vi "Settings Dialog.vi"(8 "error in (no error)":errorcluster, 11 "Settings in":T5={"Support"={"Save Configuration"={"Log File Base Path"=path "", "TDMS File Reference"=refnum, "Reset"=FALSE, "Wait"=0.0, "Start Time"=0.0, "Update Rate"=1, "Channel Names"=[], "System Preset"=variant}, "LOG Configuration"={"LOG REF"=refnum, "Writer Queue"=refnum, "Log Path"=path "", "LOG"=FALSE}, "ALARM Configuration"={"LOG REF"=refnum, "Writer Queue"=refnum, "Log Path"=path "", "UPS standby"=FALSE, "status code"=5001, "SP"=[], "Over Sens Status"=[]}, "User Details"=[], "Radome Type"="", "Timer Configuration"={"Wait"=0.0, "Next Step"="", "Writer Queue"=refnum, "Reset"=FALSE, "VISA resource"="", "Status"=[], "Valve Time"=[], "Timer queue"=refnum, "Current valve"=0, "Enable"=FALSE}}, "Process"={"Test Configuration"={"current Step"=0, "Wait"=0.0, "Next Step"="", "Writer Queue"=refnum, "Reset"=FALSE, "SEQ Time"=0, "General Reset"=FALSE, "Cycles"=0, "Status"=[], "Ready"=[], "Backward"=FALSE, "Current SP"=[], "System Preset"={"Test Configuration"={"Cycles"=0, "Z Up"=0.0, "SP List"=[], "Operator"="", "Point Delay"=0, "Z Up 2"=0.0, "Cleaning In"=0.0, "Cleaning Out"=0.0, "Cleaning Cycles"=0}, "Test_Start_date"=""}, "Test Type"=enum."Calibration", "Sample Count"=0, "Local Queues"={"Cycles queue"=refnum, "Step queue"=refnum, "RES Queue"=refnum, "Clean queue"=refnum, "PS Scan queue"=refnum}, "current Clean"=0, "PS Measure Plan"=[]}}, "Report Configuration"={"Test Setting"={"Test_Num"=0, "Test_ID"=0, "Proc_ID"=0, "Max Force"=0.0, "User"="", "SN"="", "Date"=""}, "Measurements"=[], "LOG REF"=refnum, "Report Template"=path "", "Save Report path"=path "", "Data File Path"=path "", "Popup Dialog"=FALSE}, "History Data"={"Tests"=[], "Test Name"=""}, "Motor Configuration"={"Tango HW"={"VISA resource"="", "Baud Rate (115200)"=2, "lAnInterfaceType"=0, "bAShowProt"=15}, "Writer Queue"=refnum, "Status"=FALSE, "Abs Position"=[], "Axis Velocity"={"dX"=0.0, "dY"=0.0, "dZ"=0.0, "dA"=0.0}, "acceleration "=0.0, "Z direction"=enum."Up", "Position Mode"="", "plLSID"=0}, "PalmSense  Configuration"={"PalmSens.lvclass"=refnum, "Writer Queue"=refnum, "Enable"=FALSE, "Is Measuring Ref"=refnum, "Method"={"Name"="", "Method Ref"=variant}, "PS Live Curve Result"=refnum}, "Hiden Scanner Resources"={"Link"={"Connection"=enum."USB", "Host or IP address (TCP/IP)"="", "Port (Serial/USB)"="COM1"}, "VISA resource"="", "Writer Queue"=refnum, "Status"=FALSE}, "MFC Configuration"={"MFC Definition"={"MFC Port"="", "MFC Enable"=TRUE, "Baud Rate"=0, "Interface type"=enum."RS-485", "Address"=0}, "Set Point Options"={"Setpoint Value"=0.0, "Mass Flow EU 2"="", "Setpoint Source"="", "Valve Mode"=""}, "Writer Queue"=refnum, "Enable"=FALSE, "Update Rate"=0, "MRC Chamber Enable"=FALSE, "Selected Gas"="", "Address String"=""}, "Pump Configuration"={"Pump  name"=[], "Writer Queue"=refnum, "Pump Info"={"Pump Type"="", "Speed"=0, "Direction"=0, "Running"=FALSE}, "Current Pump Name"="", "Wait"=0.0, "Next Step"="", "Reset"=FALSE}} {"Pump Configuration"."Pump Info"."Direction" items=["CW", "CCW"]; "Pump Configuration"."Pump Info"."Speed" format="%03.0f"; "MFC Configuration"."Set Point Options"."Setpoint Value" min=0.0 max=0.62495 format="%.5f"; "Process"."Test Configuration"."PS Measure Plan" items=["Pretreatment settings (PS)", "Linear Sweep Voltammetry (LSV)", "Differential Pulse Voltammetry (DPV)", "Cyclic Voltammetry (CV)", "Chronoamperometry (CA)", "Chronopotentiometry (CP)", "El Imp Spectroscopy (EIS)"]; "Process"."Test Configuration"."System Preset"."Test Configuration"."SP List" format="%#.1g"; "Support"."Save Configuration"."Update Rate" min=1 max=10 step=1}) -> (0 "error out":errorcluster, 1 "Cancelled?":bool, 2 "UI Refresh Needed?":bool, 3 "Settings out":T5={"Support"={"Save Configuration"={"Log File Base Path"=path "", "TDMS File Reference"=refnum, "Reset"=FALSE, "Wait"=0.0, "Start Time"=0.0, "Update Rate"=1, "Channel Names"=[], "System Preset"=variant}, "LOG Configuration"={"LOG REF"=refnum, "Writer Queue"=refnum, "Log Path"=path "", "LOG"=FALSE}, "ALARM Configuration"={"LOG REF"=refnum, "Writer Queue"=refnum, "Log Path"=path "", "UPS standby"=FALSE, "status code"=5001, "SP"=[], "Over Sens Status"=[]}, "User Details"=[], "Radome Type"="", "Timer Configuration"={"Wait"=0.0, "Next Step"="", "Writer Queue"=refnum, "Reset"=FALSE, "VISA resource"="", "Status"=[], "Valve Time"=[], "Timer queue"=refnum, "Current valve"=0, "Enable"=FALSE}}, "Process"={"Test Configuration"={"current Step"=0, "Wait"=0.0, "Next Step"="", "Writer Queue"=refnum, "Reset"=FALSE, "SEQ Time"=0, "General Reset"=FALSE, "Cycles"=0, "Status"=[], "Ready"=[], "Backward"=FALSE, "Current SP"=[], "System Preset"={"Test Configuration"={"Cycles"=0, "Z Up"=0.0, "SP List"=[], "Operator"="", "Point Delay"=0, "Z Up 2"=0.0, "Cleaning In"=0.0, "Cleaning Out"=0.0, "Cleaning Cycles"=0}, "Test_Start_date"=""}, "Test Type"=enum."Calibration", "Sample Count"=0, "Local Queues"={"Cycles queue"=refnum, "Step queue"=refnum, "RES Queue"=refnum, "Clean queue"=refnum, "PS Scan queue"=refnum}, "current Clean"=0, "PS Measure Plan"=[]}}, "Report Configuration"={"Test Setting"={"Test_Num"=0, "Test_ID"=0, "Proc_ID"=0, "Max Force"=0.0, "User"="", "SN"="", "Date"=""}, "Measurements"=[], "LOG REF"=refnum, "Report Template"=path "", "Save Report path"=path "", "Data File Path"=path "", "Popup Dialog"=FALSE}, "History Data"={"Tests"=[], "Test Name"=""}, "Motor Configuration"={"Tango HW"={"VISA resource"="", "Baud Rate (115200)"=2, "lAnInterfaceType"=0, "bAShowProt"=15}, "Writer Queue"=refnum, "Status"=FALSE, "Abs Position"=[], "Axis Velocity"={"dX"=0.0, "dY"=0.0, "dZ"=0.0, "dA"=0.0}, "acceleration "=0.0, "Z direction"=enum."Up", "Position Mode"="", "plLSID"=0}, "PalmSense  Configuration"={"PalmSens.lvclass"=refnum, "Writer Queue"=refnum, "Enable"=FALSE, "Is Measuring Ref"=refnum, "Method"={"Name"="", "Method Ref"=variant}, "PS Live Curve Result"=refnum}, "Hiden Scanner Resources"={"Link"={"Connection"=enum."USB", "Host or IP address (TCP/IP)"="", "Port (Serial/USB)"="COM1"}, "VISA resource"="", "Writer Queue"=refnum, "Status"=FALSE}, "MFC Configuration"={"MFC Definition"={"MFC Port"="", "MFC Enable"=TRUE, "Baud Rate"=0, "Interface type"=enum."RS-485", "Address"=0}, "Set Point Options"={"Setpoint Value"=0.0, "Mass Flow EU 2"="", "Setpoint Source"="", "Valve Mode"=""}, "Writer Queue"=refnum, "Enable"=FALSE, "Update Rate"=0, "MRC Chamber Enable"=FALSE, "Selected Gas"="", "Address String"=""}, "Pump Configuration"={"Pump  name"=[], "Writer Queue"=refnum, "Pump Info"={"Pump Type"="", "Speed"=0, "Direction"=0, "Running"=FALSE}, "Current Pump Name"="", "Wait"=0.0, "Next Step"="", "Reset"=FALSE}} {"Pump Configuration"."Pump Info"."Direction" items=["CW", "CCW"]; "Pump Configuration"."Pump Info"."Speed" format="%03.0f"; "MFC Configuration"."Set Point Options"."Setpoint Value" min=0.0 max=0.62495 format="%.5f"; "Process"."Test Configuration"."PS Measure Plan" items=["Pretreatment settings (PS)", "Linear Sweep Voltammetry (LSV)", "Differential Pulse Voltammetry (DPV)", "Cyclic Voltammetry (CV)", "Chronoamperometry (CA)", "Chronopotentiometry (CP)", "El Imp Spectroscopy (EIS)"]; "Process"."Test Configuration"."System Preset"."Test Configuration"."SP List" format="%#.1g"; "Support"."Save Configuration"."Update Rate" min=1 max=10 step=1})   [LabVIEW 2020, in "Settings.lvlib"]
doc: "Dialog for selecting user specified settings."
uses:
  Settings.lvlib
  Settings.ctl
  <instrlib>/PalmSens SDK for LabVIEW 5.10/PalmSens/PalmSens.lvclass
  Logging/Save Configuration.ctl
  LOG/LOG Configuration.ctl
  support/Message Queue/Message Cluster.ctl
  ALARM/ALARM Configuration.ctl
  Valve Control/AM Configuration.ctl
  Test Driver/Test Driver Configuration.ctl
  Test Driver/System Preset.ctl
  Test Driver/Test Type.ctl
  Report/REP Configuration.ctl
  Report/Test Setting.ctl
  MOTOR/PS Hardware Configuration.ctl
  DMM/PalmSense Hardware Configuration.ctl
  Hiden Scanner/Scanner Hardware Configuration.ctl
  MRC/MRC Configuration.ctl
  WM Pump/Pump Hardware Configuration.ctl
  support/PCT FGV CMD.ctl
  <vilib>/Utility/file.llb/Write Delimited Spreadsheet (DBL).vi
  <vilib>/Utility/file.llb/Read Delimited Spreadsheet (DBL).vi
  <vilib>/Analysis/1siggen.llb/Ramp Pattern by Delta.vi
  <vilib>/gmath/interp.llb/Create Mesh Grid (2D) (x,y arrays).vi
  <vilib>/Utility/xml.llb/Write to XML File(string).vi
  <vilib>/Analysis/NI_AALBase.lvlib
  <vilib>/gmath/NI_Gmath.lvlib
  Logging/SAVE.lvlib
  support/Message Queue/Message Queue.lvlib
  LOG/LOG.lvlib
  ALARM/QCT ALARM.lvlib
  Report/Report.lvlib
  MOTOR/MOTOR.lvlib
  Test Driver/Test Driver.lvlib
  DMM/PalmSens.lvlib
  Hiden Scanner/Hiden Scanner.lvlib
  Valve Control/Valve Control.lvlib
  MRC/MRC Module.lvlib
  WM Pump/Pump.lvlib
panel:
  in  "OK Button":bool
  in  "Cancel Button":bool
  out "Tab Control":enum32{"Administrator", "System", "Test"}(tab)
  in  "Tango XYZ":T1={"Position Mode"="Absolute", "XYZ Velocity"=0.0}
  in  "PS Measure Plan":u16[](array[ring]) items=["Pretreatment settings (PS)", "Linear Sweep Voltammetry (LSV)", "Differential Pulse Voltammetry (DPV)", "Cyclic Voltammetry (CV)", "Chronoamperometry (CA)", "Chronopotentiometry (CP)", "El Imp Spectroscopy (EIS)"]
  in  "Hiden Scan Details":dbl[][](array[numeric])=[[28.0, 28.0]]
  in  "PS Measure Type List":u16(ring)=1 items=["Pretreatment settings (PS)", "Linear Sweep Voltammetry (LSV)", "Differential Pulse Voltammetry (DPV)", "Cyclic Voltammetry (CV)", "Chronoamperometry (CA)", "Chronopotentiometry (CP)", "El Imp Spectroscopy (EIS)"]
  in  "Log File Path":path
  in  "Save Report Path":path
  in  "Report Template":path
  in  "Hiden Input details":T2={"Input device"="Faraday", "Autorange High"=-7, "Autorange Low"=-7, "Start range"=-7, "Dwell (%)"=100, "Settle (%)"=100, "Dwell is ms?"=FALSE, "Settle is ms?"=FALSE}
  out "Technician":string
  in  "Main Axis":enum32{"X Axis", "Y Axis"}(radio)
  in  "Square":cluster{"Start":dbl, "End":dbl, "delta":dbl} caption="Square / Radius SET"
  in  "Circle":cluster{"Points N":dbl, "M Point":dbl[]} caption="Y Start-Stop Point"
  in  "Shape Type":T3(ring)
  in  "Test Configuration":T4 {"SP List" format="%#.1g"}
  in  "Tests List":string(combo)
  in  "Save Test":bool
  out "XY Graph":cluster{"X":dbl[], "Y":dbl[]}[](graph)
  in  "Radio Buttons":enum32{"Administrator", "System", "Test"}(radio)=enum."System"
  out "power":bool
  # "Non visible portion of dialog (needed for connector pane)."
  # "TANGO XYZ"
  # "X"
  # "Y"
  # "Cycles"
  # "Point Delay"
  # "Up"
  # "Down"
  # "Z Axes"
  # "#C"
  # "In"
  # "Out"
  # "Cleaning [sec]"
  # "X"
  # "Y"
  # "Cycles"
  # "Point Delay"
  # "Up"
  # "Down"
  # "Z Axes"
  # "#C"
  # "In"
  # "Out"
  # "Cleaning [sec]"
  # "X"
  # "Y"
  # "Cycles"
  # "Point Delay"
  # "Up"
  # "Down"
  # "Z Axes"
  # "#C"
  # "In"
  # "Out"
  # "Cleaning [sec]"
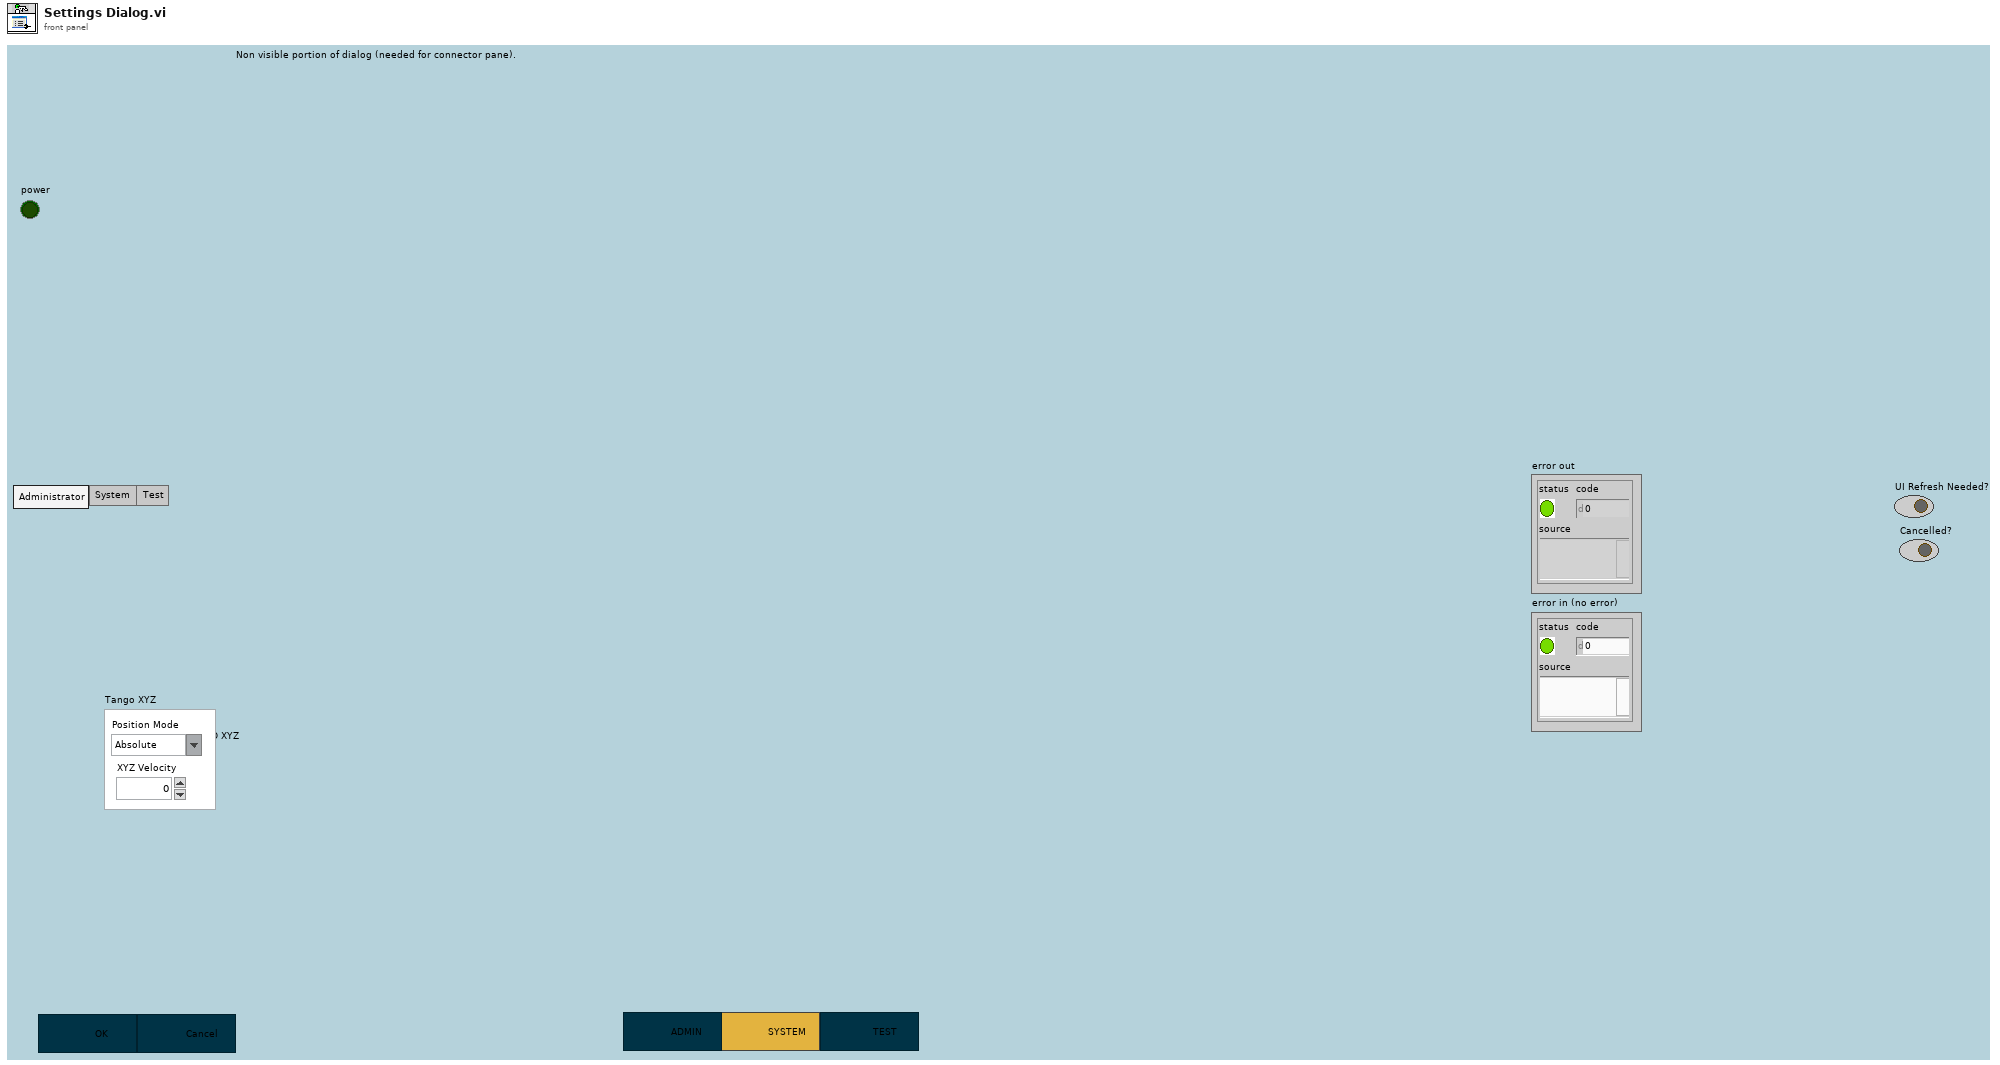
[diagram p1: front panel]
types:
  T1 = cluster{"Position Mode":string, "XYZ Velocity":dbl}
  T2 = cluster{"Input device":string, "Autorange High":i16, "Autorange Low":i16, "Start range":i16, "Dwell (%)":u16, "Settle (%)":u16, "Dwell is ms?":bool, "Settle is ms?":bool}
  T3 = enum16{"Circle", "Square", "Ramp", "Mesh", "Line"}
  T4 = cluster{"Cycles":i32, "Z Up":dbl, "SP List":dbl[][], "Operator":string, "Point Delay":i32, "Z Up 2":dbl, "Cleaning In":dbl, "Cleaning Out":dbl, "Cleaning Cycles":i32}
  T5 = typedef "Settings.lvlib/Settings.ctl" = cluster{"Support":cluster{"Save Configuration":T6, "LOG Configuration":T7, "ALARM Configuration":T8, "User Details":string[], "Radome Type":string, "Timer Configuration":T9}, "Process":cluster{"Test Configuration":T10}, "Report Configuration":T13, "History Data":cluster{"Tests":string[][], "Test Name":string}, "Motor Configuration":T15, "PalmSense  Configuration":T16, "Hiden Scanner Resources":T17, "MFC Configuration":T18, "Pump Configuration":T19}
  T6 = typedef "SAVE.lvlib/Save Configuration.ctl" = cluster{"Log File Base Path":path, "TDMS File Reference":refnum<k34>, "Reset":bool, "Wait":dbl, "Start Time":dbl, "Update Rate":u16, "Channel Names":string[], "System Preset":variant}
  T7 = typedef "LOG.lvlib/LOG Configuration.ctl" = cluster{"LOG REF":refnum<vi>, "Writer Queue":refnum<queue>, "Log Path":path, "LOG":bool}
  T8 = typedef "QCT ALARM.lvlib/ALARM Configuration.ctl" = cluster{"LOG REF":refnum<vi>, "Writer Queue":refnum<queue>, "Log Path":path, "UPS standby":bool, "status code":i32, "SP":dbl[], "Over Sens Status":dbl[]}
  T9 = typedef "Valve Control.lvlib/AM Configuration.ctl" = cluster{"Wait":dbl, "Next Step":string, "Writer Queue":refnum<queue>, "Reset":bool, "VISA resource":refnum<visa-resource-name>, "Status":bool[], "Valve Time":dbl[], "Timer queue":refnum<queue>, "Current valve":i32, "Enable":bool}
  T10 = typedef "Test Driver.lvlib/Test Driver Configuration.ctl" = cluster{"current Step":i32, "Wait":dbl, "Next Step":string, "Writer Queue":refnum<queue>, "Reset":bool, "SEQ Time":i32, "General Reset":bool, "Cycles":i32, "Status":bool[], "Ready":bool[], "Backward":bool, "Current SP":dbl[], "System Preset":T11, "Test Type":T12, "Sample Count":i32, "Local Queues":cluster{"Cycles queue":refnum<queue>, "Step queue":refnum<queue>, "RES Queue":refnum<queue>, "Clean queue":refnum<queue>, "PS Scan queue":refnum<queue>}, "current Clean":i32, "PS Measure Plan":u16[]}
  T11 = typedef "System Preset.ctl" = cluster{"Test Configuration":cluster{"Cycles":i32, "Z Up":dbl, "SP List":dbl[][], "Operator":string, "Point Delay":i32, "Z Up 2":dbl, "Cleaning In":dbl, "Cleaning Out":dbl, "Cleaning Cycles":i32}, "Test_Start_date":string}
  T12 = typedef "Test Driver.lvlib/Test Type.ctl" = enum16{"Calibration", "Test"}
  T13 = typedef "Report.lvlib/REP Configuration.ctl" = cluster{"Test Setting":T14, "Measurements":string[][], "LOG REF":refnum<vi>, "Report Template":path, "Save Report path":path, "Data File Path":path, "Popup Dialog":bool}
  T14 = typedef "Report.lvlib/Test Setting.ctl" = cluster{"Test_Num":i32, "Test_ID":i32, "Proc_ID":i32, "Max Force":dbl, "User":string, "SN":string, "Date":string}
  T15 = typedef "MOTOR.lvlib/PS Hardware Configuration.ctl" = cluster{"Tango HW":cluster{"VISA resource":refnum<visa-resource-name>, "Baud Rate (115200)":i32, "lAnInterfaceType":i32, "bAShowProt":i32}, "Writer Queue":refnum<queue>, "Status":bool, "Abs Position":i32[], "Axis Velocity":cluster{"dX":dbl, "dY":dbl, "dZ":dbl, "dA":dbl}, "acceleration ":dbl, "Z direction":enum16{"Up", "Down"}, "Position Mode":string, "plLSID":i32}
  T16 = typedef "PalmSens.lvlib/PalmSense Hardware Configuration.ctl" = cluster{"PalmSens.lvclass":refnum<class "PalmSens.lvclass">, "Writer Queue":refnum<queue>, "Enable":bool, "Is Measuring Ref":refnum<vi>, "Method":cluster{"Name":string, "Method Ref":variant}, "PS Live Curve Result":refnum<vi>}
  T17 = typedef "Hiden Scanner.lvlib/Scanner Hardware Configuration.ctl" = cluster{"Link":cluster{"Connection":enum16{"Serial", "TCP/IP", "USB"}, "Host or IP address (TCP/IP)":string, "Port (Serial/USB)":string}, "VISA resource":refnum<visa-resource-name>, "Writer Queue":refnum<queue>, "Status":bool}
  T18 = typedef "MRC Module.lvlib/MRC Configuration.ctl" = cluster{"MFC Definition":cluster{"MFC Port":refnum<visa-resource-name>, "MFC Enable":bool, "Baud Rate":i32, "Interface type":enum32{"RS-485", "RS-232"}, "Address":i32}, "Set Point Options":cluster{"Setpoint Value":dbl, "Mass Flow EU 2":string, "Setpoint Source":string, "Valve Mode":string}, "Writer Queue":refnum<queue>, "Enable":bool, "Update Rate":u32, "MRC Chamber Enable":bool, "Selected Gas":string, "Address String":string}
  T19 = typedef "Pump.lvlib/Pump Hardware Configuration.ctl" = cluster{"Pump  name":refnum<visa-resource-name>[], "Writer Queue":refnum<queue>, "Pump Info":cluster{"Pump Type":string, "Speed":i32, "Direction":u16, "Running":bool}, "Current Pump Name":refnum<visa-resource-name>, "Wait":dbl, "Next Step":string, "Reset":bool}
  T20 = typedef "PCT FGV CMD.ctl" = enum16{"INIT", "GET", "SET"}
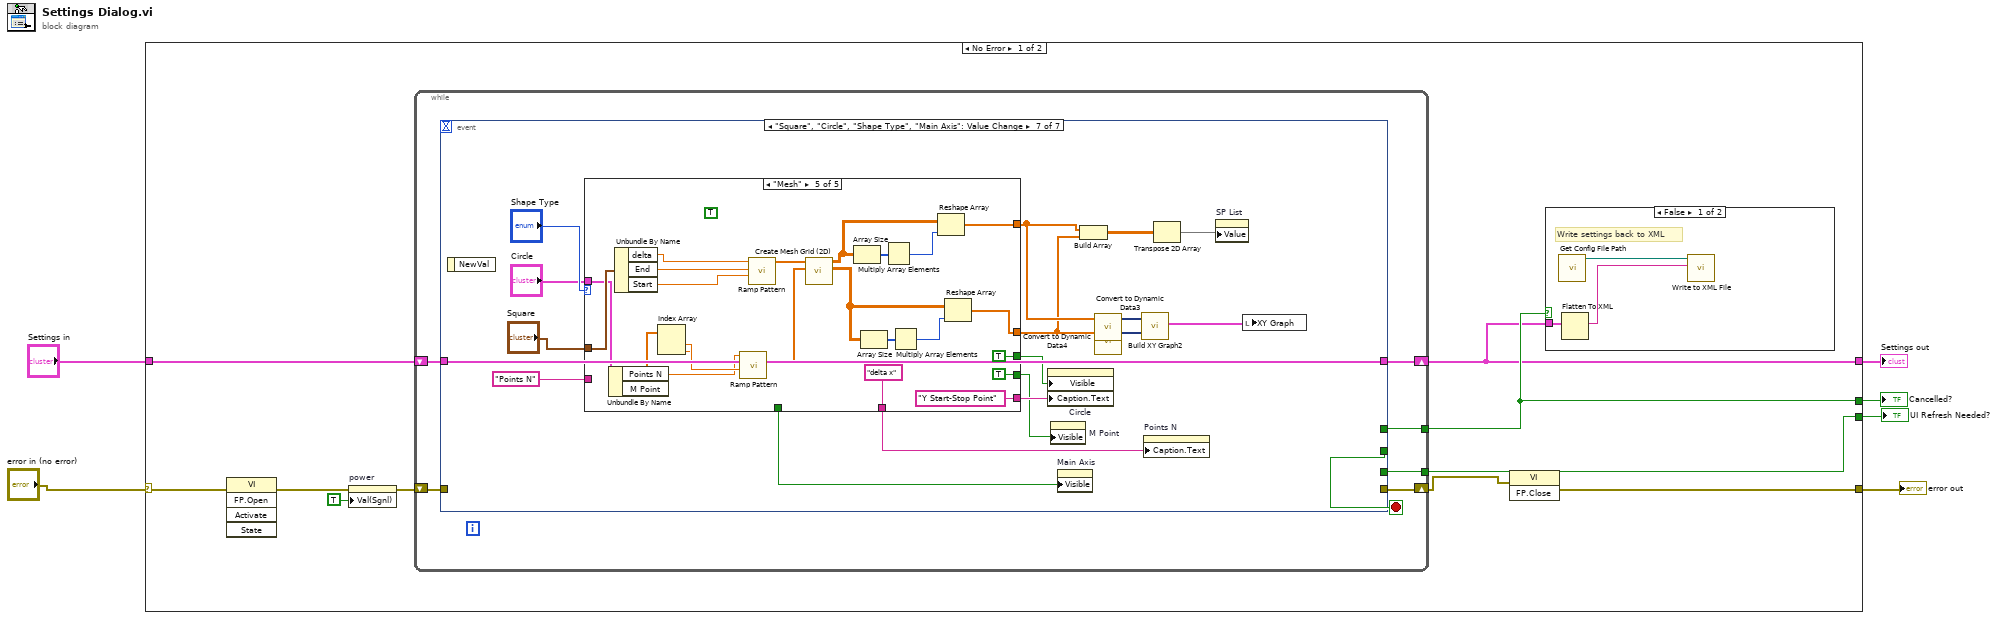
[diagram p0: block diagram]
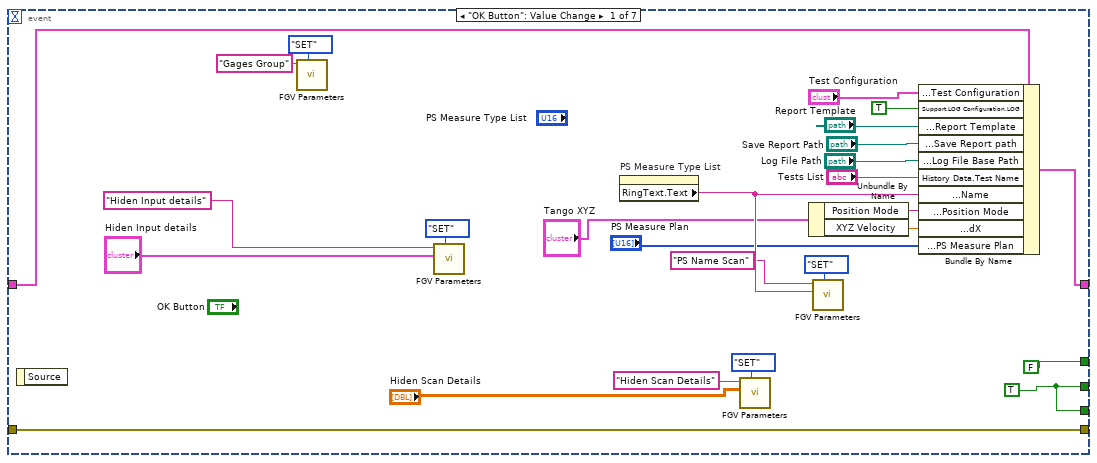
[diagram p2: hidden frame]
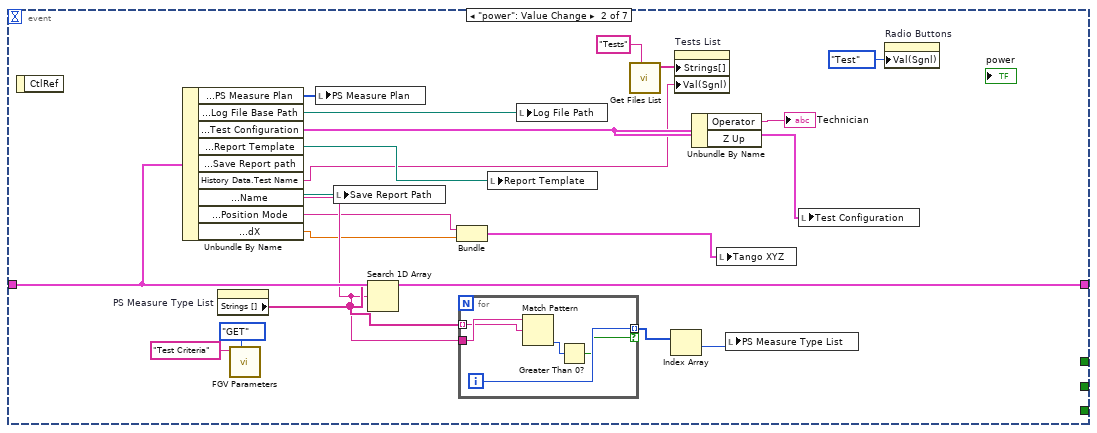
[diagram p3: hidden frame]
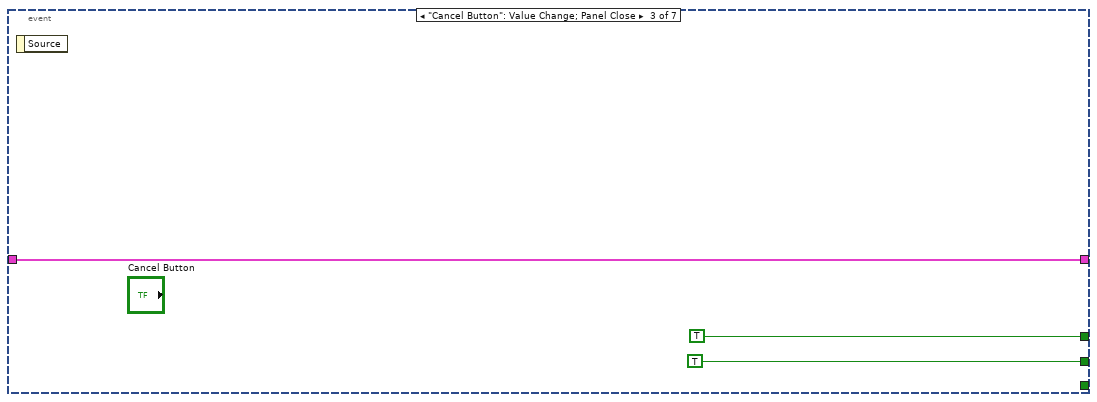
[diagram p4: hidden frame]
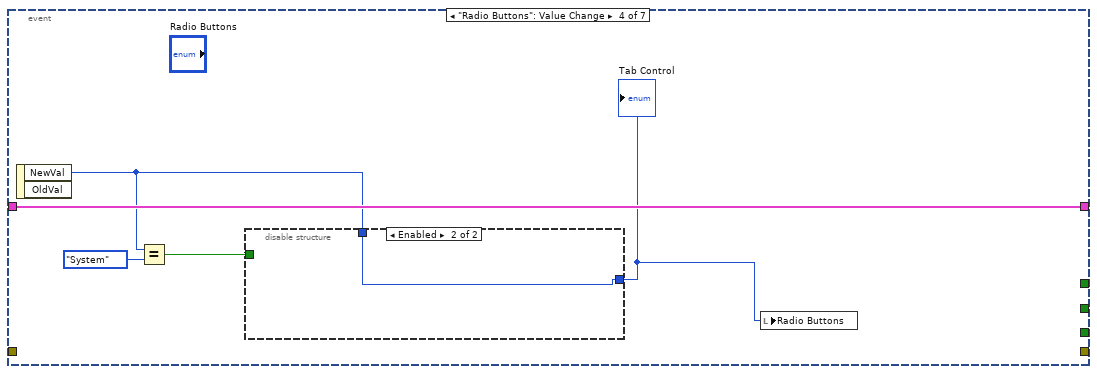
[diagram p5: hidden frame]
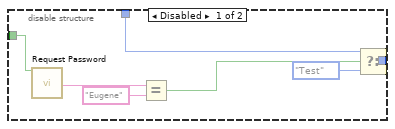
[diagram p6: hidden frame]
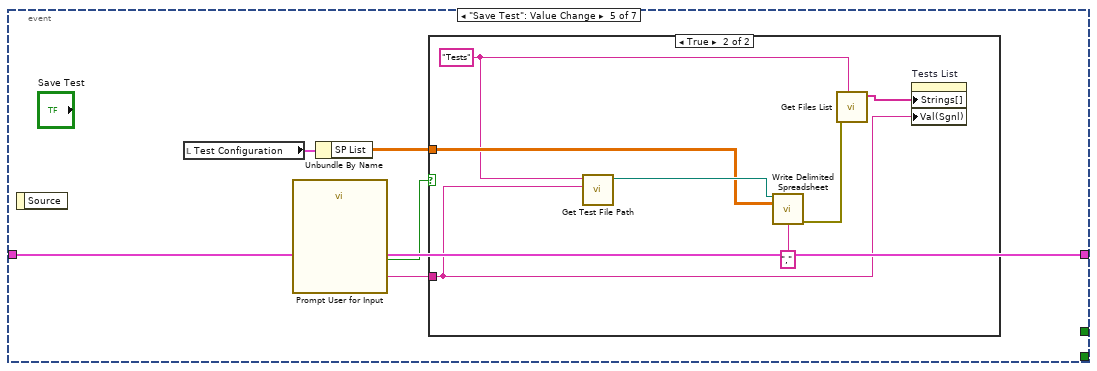
[diagram p7: hidden frame]
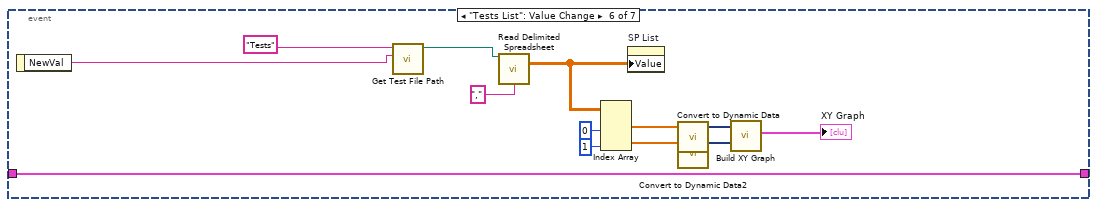
[diagram p9: hidden frame]
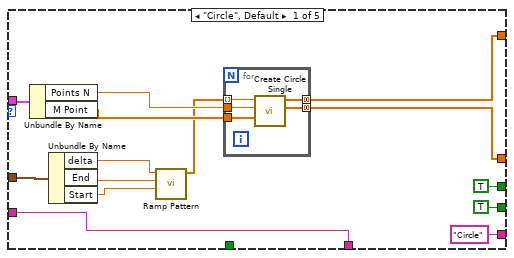
[diagram p10: hidden frame]
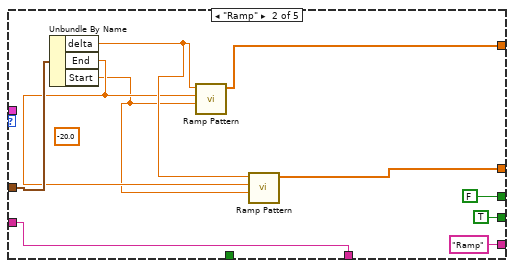
[diagram p11: hidden frame]
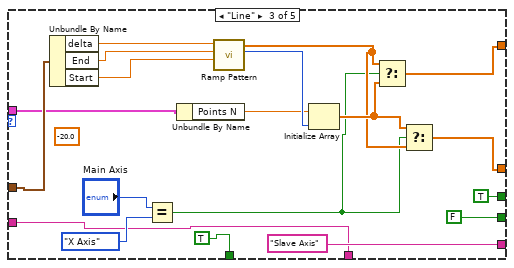
[diagram p12: hidden frame]
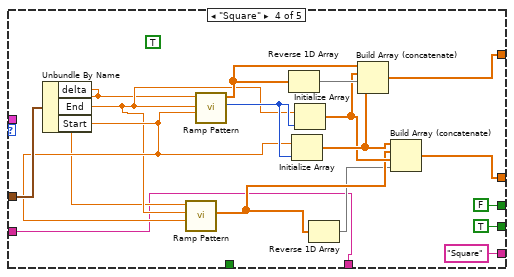
[diagram p13: hidden frame]
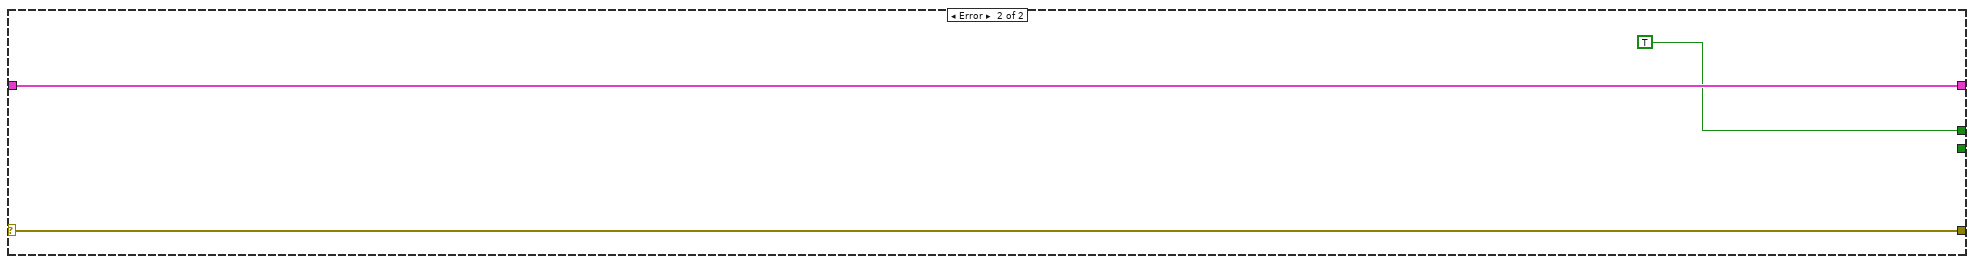
[diagram p15: hidden frame]
diagram:
  n1 = case shown="No Error" "error in (no error)" {
    selector: "error in (no error)" -> [w12 w226]
    tunnel: [w11 w226] -> w5
    tunnel: "Settings in" -> [w14 w225]
    tunnel: [w15 w225] -> w4
    tunnel: [w7 _] -> w3
    tunnel: [w16 TRUE ("UI Refresh Needed?")] -> w2
    frame No Error {
      n2 = invoke class="VI" method="FP.Open"(error in=w12) -> (error out=w10:errorcluster)  [unwired: 4 in, 4 out]
      n3 = property on="power" class="Bool (strict)"(error in=w10, "Val(Sgnl)"=TRUE ("Value (Signaling)")) -> (error out=w8:errorcluster)  [unwired: 1 in, 1 out]
      n4 = while {
        tunnel: [w19] -> w16
        shift-right: [w23] -> w15
        shift-left: w14 -> [w22]
        shift-right: [w20] -> w13
        shift-left: w8 -> [w21]
        tunnel: [w17] -> w7
        stop <- w18 stop-if-true
        n5 = event shown="[6] \"Square\", \"Circle\", \"Shape Type\", \"Main Axis\": Value Change" {
          selector: _ -> [_ _ _ _ _ _ _]
          dyn-events: _ -> [_ _ _ _ _ _ _]
          timeout: _ -> [_ _ _ _ _ _ _]
          tunnel: [w48 w69 w77 w82 w95 w115 w132] -> w23
          tunnel: w22 -> [w43 w69 w77 w82 w95 w115 w132]
          tunnel: [FALSE ("UI Refresh Needed?") _ TRUE ("UI Refresh Needed?") _ _ _ _] -> w19
          tunnel: w21 -> [w47 _ _ _ _ _ _]
          tunnel: [w47 _ _ _ _ _ _] -> w20
          tunnel: [w39 _ TRUE _ _ _ _] -> w18
          tunnel: [w39 _ _ _ _ _ _] -> w17
          event "OK Button": Value Change {
            w39 = TRUE
            n6 = event-data() -> ()  [unwired: 1 in, 1 out]
            n7 = call "FGV Parameters.vi"("CMD"=PCT_FGV_CMD."SET", "Key"="Gages Group") -> ()  [unwired: 7 in, 3 out]
            n8 = call "FGV Parameters.vi"("CMD"=PCT_FGV_CMD."SET", "input"="Hiden Input details", "Key"="Hiden Input details") -> ()  [unwired: 6 in, 3 out]
            n9 = property on="PS Measure Type List" class="Ring (strict)"() -> ("RingText.Text"=w29:string)  [unwired: 2 in, 2 out]
            n10 = call "FGV Parameters.vi"("CMD"=PCT_FGV_CMD."SET", "input"="Hiden Scan Details", "Key"="Hiden Scan Details") -> ()  [unwired: 6 in, 3 out]
            n11 = Unbundle By Name("Tango XYZ") -> ("Position Mode"=w27:string, "XYZ Velocity"=w25:dbl)
            n12 = call "FGV Parameters.vi"("CMD"=PCT_FGV_CMD."SET", "input"=w29, "Key"="PS Name Scan") -> ()  [unwired: 6 in, 3 out]
            n13 = Bundle By Name(cluster=w43, "Process.Test Configuration.System Preset.Test Configuration"="Test Configuration", "Support.LOG Configuration.LOG"=TRUE, "Report Configuration.Report Template"="Report Template", "Report Configuration.Save Report path"="Save Report Path", "Support.Save Configuration.Log File Base Path"="Log File Path", "History Data.Test Name"="Tests List", "PalmSense  Configuration.Method.Name"=w29, "Motor Configuration.Position Mode"=w27, "Motor Configuration.Axis Velocity.dX"=w25, "Process.Test Configuration.PS Measure Plan"="PS Measure Plan") -> (w48:T5)
          }
          event "power": Value Change {
            n14 = event-data() -> ()  [unwired: 1 in, 1 out]
            n15 = Unbundle By Name(w69) -> ("Process.Test Configuration.PS Measure Plan"=w50:u16[], "Support.Save Configuration.Log File Base Path"=w66:path, "Process.Test Configuration.System Preset.Test Configuration"=w62:T4, "Report Configuration.Report Template"=w68:path, "Report Configuration.Save Report path"=w67:path, "History Data.Test Name"=w59:string, "PalmSense  Configuration.Method.Name"=w57:string, "Motor Configuration.Position Mode"=w53:string, "Motor Configuration.Axis Velocity.dX"=w52:dbl)
            n16 = property on="PS Measure Type List" class="Ring (strict)"() -> ("Strings []"=w58:string[])  [unwired: 2 in, 2 out]
            n17 = call "FGV Parameters.vi"("CMD"=PCT_FGV_CMD."GET", "Key"="Test Criteria") -> ()  [unwired: 7 in, 3 out]
            n18 = local write "PS Measure Plan"(w50) -> ()
            n19 = local write "Save Report Path"(w67) -> ()
            n20 = Search 1D Array(1D array=w58, element=w57) -> ()  [unwired: 1 in, 1 out]
            n21 = Bundle("Position Mode"=w53, "dX"=w52) -> (w51:cluster{"Position Mode":string, "dX":dbl})  [unwired: 1 in]
            n22 = for {
              tunnel: w58 -> [w73] mode=indexing
              tunnel: w57 -> [w74]
              tunnel: [w72] -> w56 mode=indexing if=w70
              i -> [w72]
              n23 = Match Pattern(string=w74, regular expression=w73) -> (offset past match=w71:i32)  [unwired: 1 in, 3 out]
              n24 = Greater Than 0?(x=w71) -> (x > 0?=w70:bool)
            }
            n25 = local write "Report Template"(w68) -> ()
            n26 = local write "Log File Path"(w66) -> ()
            n27 = call "Get Files List.vi"("Folder Name"="Tests") -> ("List"=w60:string[])  [unwired: 9 in, 1 out]
            n28 = Index Array(array=w56) -> (element=w55:i32)  [unwired: 1 in]
            n29 = property on="Tests List" class="CmbBox"("Strings[]"=w60, "Val(Sgnl)"=w59) -> ()  [unwired: 2 in, 2 out]
            n30 = Unbundle By Name(w62) -> ("Operator"=→"Technician":string)  [unwired: 1 out]
            n31 = local write "Tango XYZ"(w51) -> ()
            n32 = local write "PS Measure Type List"(w55) -> ()
            n33 = local write "Test Configuration"(w62) -> ()
            n34 = property on="Radio Buttons" class="RadioBtnsControl (strict)"("Val(Sgnl)"=enum32{"Administrator", "System", "Test"}."Test" ("Value (Signaling)")) -> ()  [unwired: 2 in, 2 out]
          }
          event "Cancel Button": Value Change; Panel Close {
            n35 = event-data() -> ()  [unwired: 1 in, 1 out]
          }
          event "Radio Buttons": Value Change {
            n36 = event-data() -> ("NewVal"=w80:enum32{"Administrator", "System", "Test"})  [unwired: 1 in, 1 out]
            n37 = Equal?(x=w80, y=enum32{"System", "Test"}."System") -> (x = y?=w79:bool)
            n38 = disable-structure shown="Enabled" {
              disable-tunnel: w80 -> [w86 w90]
              disable-tunnel: w79 -> [w85 _]
              disable-tunnel: [w84 w90] -> w78
              frame Disabled {
                n39 = call "Request Password.vi"("Enable"=w85) -> ("Password"=w89:string)  [unwired: 16 in, 2 out]
                n40 = Equal?(x=w89, y="Eugene") -> (x = y?=w83:bool)
                n41 = Select(t=w86, s=w83, f=enum32{"System", "Test"}."Test" ("Radio Buttons")) -> (s? t:f=w84:u32)
              }
              frame Enabled {
              }
            }
            "Tab Control" <- w78
            n42 = local write "Radio Buttons"(w78) -> ()
          }
          event "Save Test": Value Change {
            n43 = event-data() -> ()  [unwired: 1 in, 1 out]
            n44 = local read "Test Configuration"() -> (w94:T4)
            n45 = call "Prompt User for Input"() -> ("Test Name"=w92:string, "OK"=w93:bool)  [unwired: 17 in, 1 out]
            n46 = Unbundle By Name(w94) -> ("SP List"=w91:dbl[][])
            n47 = case shown="True" w93 {
              tunnel: w92 -> [_ w96]
              tunnel: w91 -> [_ w101]
              frame False {
              }
              frame True {
                w99 = "Tests" ("Folder Name")
                n48 = call "Get Test File Path.vi"("Test Name"=w96, "Folder Name"=w99) -> ("test path"=w102:path)  [unwired: 9 in]
                n49 = call-poly <vilib>:"Write Delimited Spreadsheet.vi"("file path (dialog if empty)"=w102, "2D data"=w101, "delimiter (\\t)"="," ("delimiter (\\t)")) -> ("error out"=w98:errorcluster)  [unwired: 11 in, 1 out]
                n50 = call "Get Files List.vi"("Folder Name"=w99, "error in (no error)"=w98) -> ("List"=w97:string[])  [unwired: 8 in, 1 out]
                n51 = property on="Tests List" class="CmbBox"("Strings[]"=w97, "Val(Sgnl)"=w96) -> ()  [unwired: 2 in, 2 out]
              }
            }
          }
          event "Tests List": Value Change {
            n52 = event-data() -> ("NewVal"=w103:string)  [unwired: 1 in]
            n53 = call "Get Test File Path.vi"("Test Name"=w103, "Folder Name"="Tests") -> ("test path"=w113:path)  [unwired: 9 in]
            n54 = call-poly <vilib>:"Read Delimited Spreadsheet.vi"("file path (dialog if empty)"=w113, "delimiter (\\t)"="," ("delimiter (\\t)")) -> ("all rows"=w111:dbl[][])  [unwired: 8 in, 5 out]
            n55 = Index Array(array=w111, index (col) #1=0 ("disabled index (col)"), index (col) #2=1 ("index (col)")) -> (element #1=w108:dbl[], element #2=w106:dbl[])  [unwired: 2 in]
            n56 = property on="SP List" class="Arr (strict)"("Value"=w111) -> ()  [unwired: 2 in, 2 out]
            n57 = call "Convert to Dynamic Data"("Array"=w108) -> ("Dynamic Data Type"=w107:dynamicdata)  [unwired: 3 in]
            n58 = call "Convert to Dynamic Data2"("Array"=w106) -> ("Dynamic Data Type"=w105:dynamicdata)  [unwired: 3 in]
            n59 = call "Build XY Graph"("Y Input"=w105, "X Input"=w107) -> ("XY Graph"=→"XY Graph":cluster{"X":dbl[], "Y":dbl[]}[])  [unwired: 8 in, 1 out]
          }
          event "Square", "Circle", "Shape Type", "Main Axis": Value Change {
            n60 = event-data() -> ()  [unwired: 1 in, 1 out]
            n61 = case shown="\"Mesh\"" "Shape Type" {
              tunnel: [w143 w160 w168 w194 w211] -> w125
              tunnel: [w142 w161 w167 w189 w207] -> w122
              tunnel: "Circle" -> [w146 _ w175 _ w203]
              tunnel: "Square" -> [w141 w159 w180 w188 w220]
              tunnel: ["Circle" "Ramp" "Slave Axis" "Square" "Y Start-Stop Point"] -> w121
              tunnel: [TRUE TRUE FALSE TRUE TRUE] -> w120
              tunnel: [TRUE FALSE TRUE FALSE TRUE] -> w119
              tunnel: [_ _ TRUE _ _] -> w118
              tunnel: [w133 w152 w162 w181 "delta x" ("Caption.Text")] -> w117
              tunnel: "Points N" ("Caption.Text") -> [w133 w152 w162 w181 _]
              frame "Circle", Default {
                n62 = Unbundle By Name(w146) -> ("Points N"=w145:dbl, "M Point"=w144:dbl[])
                n63 = Unbundle By Name(w141) -> ("delta"=w140:dbl, "End"=w139:dbl, "Start"=w138:dbl)
                n64 = call-poly <vilib>:"Ramp Pattern.vi"("start"=w138, "end"=w139, "delta"=w140) -> ("Ramp Pattern"=w137:dbl[])  [unwired: 6 in, 2 out]
                n65 = for {
                  tunnel: w137 -> [w147] mode=indexing
                  tunnel: w145 -> [w151]
                  tunnel: [w150] -> w143 mode=concatenating
                  tunnel: [w149] -> w142 mode=concatenating
                  tunnel: w144 -> [w148]
                  n66 = call "Create Circle Single.vi"("M Point"=w148, "Points N"=w151, "Radius"=w147) -> ("Y"=w149:dbl[], "X"=w150:dbl[])  [unwired: 7 in]
                }
              }
              frame "Ramp" {
                (unwired) -20.0 ("start")
                n67 = Unbundle By Name(w159) -> ("delta"=w158:dbl, "End"=w157:dbl, "Start"=w156:dbl)
                n68 = call-poly <vilib>:"Ramp Pattern.vi"("start"=w156, "end"=w157, "delta"=w158) -> ("Ramp Pattern"=w160:dbl[])  [unwired: 6 in, 2 out]
                n69 = call-poly <vilib>:"Ramp Pattern.vi"("start"=w156, "end"=w157, "delta"=w158) -> ("Ramp Pattern"=w161:dbl[])  [unwired: 6 in, 2 out]
              }
              frame "Line" {
                (unwired) -20.0 ("start")
                n70 = Unbundle By Name(w180) -> ("delta"=w179:dbl, "End"=w178:dbl, "Start"=w177:dbl)
                n71 = Equal?(x="Main Axis", y=enum32{"X Axis", "Y Axis"}."X Axis" ("Main Axis")) -> (x = y?=w169:bool)
                n72 = Unbundle By Name(w175) -> ("Points N"=w174:dbl)
                n73 = call-poly <vilib>:"Ramp Pattern.vi"("start"=w177, "end"=w178, "delta"=w179) -> ("samples"=w176:i32, "Ramp Pattern"=w170:dbl[])  [unwired: 6 in, 1 out]
                n74 = Initialize Array(w174, w176) -> (w171:dbl[])
                n75 = Select(t=w170, s=w169, f=w171) -> (s? t:f=w168:dbl[])
                n76 = Select(t=w171, s=w169, f=w170) -> (s? t:f=w167:dbl[])
              }
              frame "Square" {
                (unwired) TRUE ("reset phase")
                n77 = Unbundle By Name(w188) -> ("delta"=w185:dbl, "End"=w186:dbl, "Start"=w187:dbl)
                n78 = call-poly <vilib>:"Ramp Pattern.vi"("start"=w187, "end"=w186, "delta"=w185) -> ("Ramp Pattern"=w191:dbl[])  [unwired: 6 in, 2 out]
                n79 = call-poly <vilib>:"Ramp Pattern.vi"("start"=w187, "end"=w186, "delta"=w185) -> ("samples"=w195:i32, "Ramp Pattern"=w197:dbl[])  [unwired: 6 in, 1 out]
                n80 = Reverse 1D Array(array=w197) -> (reversed array=w196:dbl[])
                n81 = Initialize Array(w187, w195) -> (w193:dbl[])
                n82 = Initialize Array(w186, w195) -> (w192:dbl[])
                n83 = Reverse 1D Array(array=w191) -> (reversed array=w190:dbl[])
                n84 = Build Array (concatenate)(w197, w192, w196, w193) -> (w194:dbl[])
                n85 = Build Array (concatenate)(w193, w191, w192, w190) -> (w189:dbl[])
              }
              frame "Mesh" {
                (unwired) TRUE ("reset phase")
                n86 = Unbundle By Name(w203) -> ("Points N"=w198:dbl, "M Point"=w202:dbl[])
                n87 = Unbundle By Name(w220) -> ("delta"=w217:dbl, "End"=w218:dbl, "Start"=w219:dbl)
                n88 = Index Array(array=w202) -> (element #1=w201:dbl, element #2=w200:dbl)  [unwired: 2 in]
                n89 = call-poly <vilib>:"Ramp Pattern.vi"("start"=w201, "end"=w200, "delta"=w198) -> ("Ramp Pattern"=w215:dbl[])  [unwired: 6 in, 2 out]
                n90 = call-poly <vilib>:"Ramp Pattern.vi"("start"=w219, "end"=w218, "delta"=w217) -> ("Ramp Pattern"=w216:dbl[])  [unwired: 6 in, 2 out]
                n91 = call-poly <vilib>:"Create Mesh Grid (2D).vi"("y domain"=w215, "x domain"=w216) -> ("Y"=w208:dbl[][], "X"=w214:dbl[][])  [unwired: 7 in, 1 out]
                n92 = Array Size(array=w214) -> (size(s)=w213:i32[])
                n93 = Array Size(array=w208) -> (size(s)=w209:i32[])
                n94 = Multiply Array Elements(1:w213) -> (0:w212:i32)
                n95 = Multiply Array Elements(1:w209) -> (0:w210:i32)
                n96 = Reshape Array(w214, w212) -> (w211:dbl[])
                n97 = Reshape Array(w208, w210) -> (w207:dbl[])
              }
            }
            n98 = property on="Circle" class="Clust (strict)"("Visible"=w119, "Caption.Text"=w121) -> ()  [unwired: 2 in, 2 out]
            n99 = property on="M Point" class="Arr (strict)"("Visible"=w120) -> ()  [unwired: 2 in, 2 out]
            n100 = property on="Main Axis" class="RadioBtnsControl (strict)"("Visible"=w118) -> ()  [unwired: 2 in, 2 out]
            n101 = Build Array(w125, w122) -> (w124:dbl[][])
            n102 = call "Convert to Dynamic Data3"("Array"=w125) -> ("Dynamic Data Type"=w131:dynamicdata)  [unwired: 3 in]
            n103 = call "Convert to Dynamic Data4"("Array"=w122) -> ("Dynamic Data Type"=w130:dynamicdata)  [unwired: 3 in]
            n104 = call "Build XY Graph2"("Y Input"=w130, "X Input"=w131) -> ("XY Graph"=w129:cluster{"X":dbl[], "Y":dbl[]}[])  [unwired: 8 in, 1 out]
            n105 = property on="Points N" class="DigNum (strict)"("Caption.Text"=w117) -> ()  [unwired: 2 in, 2 out]
            n106 = Transpose 2D Array(2D array=w124) -> (transposed array=w123:dbl[][])
            n107 = property on="SP List" class="Arr (strict)"("Value"=w123) -> ()  [unwired: 2 in, 2 out]
            n108 = local write "XY Graph"(w129) -> ()
          }
        }
      }
      n109 = invoke class="VI" method="FP.Close"(error in=w13) -> (error out=w11:errorcluster)  [unwired: 2 in, 2 out]
      n110 = case shown="False" w16 {
        tunnel: w15 -> [w222 _]
        frame False {
          # "Write settings back to XML"
          n111 = call "Get Config File Path.vi"() -> ("XML File Path"=w223:path)  [unwired: 10 in, 1 out]
          n112 = Flatten To XML(6:w222) -> (2:w221:string)
          n113 = call-poly <vilib>:"Write to XML File.vi"("XML Input"=w221, "XML File Path"=w223) -> ()  [unwired: 7 in, 3 out]
        }
        frame True {
        }
      }
    }
    frame Error {
    }
  }
  "UI Refresh Needed?" <- w3
  "error out" <- w5
  "Settings out" <- w4
  "Cancelled?" <- w2
